vi "CTL_Pump Logic.vi"(7 "Pump CtlRef In":T1, 9 "Fill Cmd":bool, 10 "Drain Cmd":bool) -> (1 "Fill Out":bool, 2 "Drain Out":bool, 3 "Err":bool, 4 "Flow Rate":dbl, 5 "Run Btn":bool)   [LabVIEW 2024]
uses:
  Control Definitions/Def PumpCtlRefs.ctl
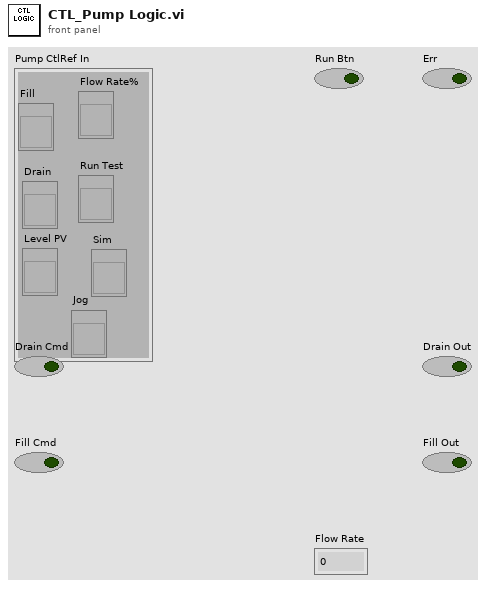
[diagram p1: front panel]
types:
  T1 = typedef "Def PumpCtlRefs.ctl" = cluster{"Fill ":refnum<vi>, "Drain":refnum<vi>, "Level PV":refnum<vi>, "Flow Rate%":refnum<vi>, "Run Test":refnum<vi>, "Sim":refnum<vi>, "Jog":refnum<vi>}
  T2 = enum8{"Enabled", "Disabled", "Disabled and Grayed Out"}
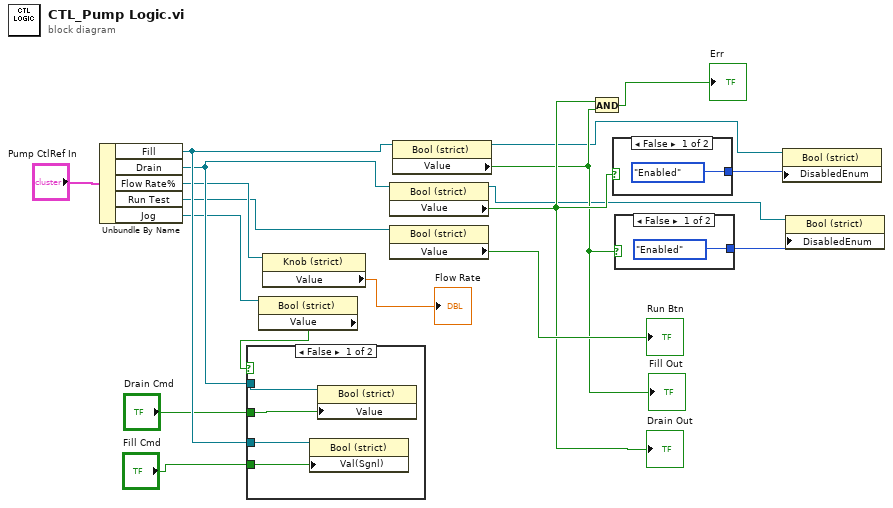
[diagram p0: block diagram]
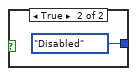
[diagram p3: hidden frame]
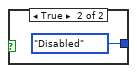
[diagram p4: hidden frame]
diagram:
  n1 = Unbundle By Name("Pump CtlRef In") -> ("Fill"=w15:refnum<vi>, "Drain"=w13:refnum<vi>, "Flow Rate%"=w4:refnum<vi>, "Run Test"=w1:refnum<vi>, "Jog"=w3:refnum<vi>)
  n2 = property on="Property Node" class="Bool (strict)"(reference=w3) -> ("Value"=w2:bool)  [unwired: 1 in, 2 out]
  n3 = case shown="False" w2 {
    tunnel: "Fill Cmd" -> [w22 _]
    tunnel: w15 -> [w21 _]
    tunnel: "Drain Cmd" -> [w20 _]
    tunnel: w13 -> [w19 _]
    frame False {
      n4 = property class="Bool (strict)"(reference=w21, "Val(Sgnl)"=w22) -> ()  [unwired: 1 in, 2 out]
      n5 = property class="Bool (strict)"(reference=w19, "Value"=w20) -> ()  [unwired: 1 in, 2 out]
    }
    frame True {
    }
  }
  n6 = property on="Property Node" class="Knob (strict)"(reference=w4) -> ("Value"=→"Flow Rate":dbl)  [unwired: 1 in, 2 out]
  n7 = property on="Property Node" class="Bool (strict)"(reference=w13) -> (reference out=w9:refnum<vi>, "Value"=w11:bool)  [unwired: 1 in, 1 out]
  "Drain Out" <- w11
  n8 = property on="Property Node" class="Bool (strict)"(reference=w1) -> ("Value"=→"Run Btn":bool)  [unwired: 1 in, 2 out]
  n9 = property on="Property Node" class="Bool (strict)"(reference=w15) -> (reference out=w8:refnum<vi>, "Value"=w10:bool)  [unwired: 1 in, 1 out]
  "Fill Out" <- w10
  n10 = And(x=w11, y=w10) -> (x .and. y?=→"Err":bool)
  n11 = case shown="False" w11 {
    tunnel: [T2."Enabled" ("Disabled") T2."Disabled" ("Disabled")] -> w6
    frame False {
    }
    frame True {
    }
  }
  n12 = case shown="False" w10 {
    tunnel: [T2."Enabled" ("Disabled") T2."Disabled" ("Disabled")] -> w7
    frame False {
    }
    frame True {
    }
  }
  n13 = property on="Property Node" class="Bool (strict)"(reference=w8, "DisabledEnum"=w6) -> ()  [unwired: 1 in, 2 out]
  n14 = property on="Property Node" class="Bool (strict)"(reference=w9, "DisabledEnum"=w7) -> ()  [unwired: 1 in, 2 out]
